vi "Create.vi"(7 "mode settings":variant, 8 "error in":errorcluster, 9 "number of default channels":i32, 10 "channel settings":variant, 11 "counter pwm input mode in":refnum<class "Counter PWM Input Mode.lvclass">) -> (0 "error out":errorcluster, 1 "channels":refnum<class "Channel.lvclass">[](array[class]), 3 "counter pwm input mode out":refnum<class "Counter PWM Input Mode.lvclass">)   [LabVIEW 2017, in "Counter PWM Input Mode.lvclass"]
uses:
  Counter PWM Input Mode.lvclass
  Channel Classes/Channel/Channel.lvclass
  Controls/counter pwm input channel settings.ctl
  Channel Classes/PWM Input Channel/Measurement Type.ctl
  f5685796-a93e-4056-970a-a8238cbbc772.vi
  Channel Classes/PWM Input Channel/PWM Input Channel.lvclass
  C:/dev/github.com/debryant/niveristand-scan-engine-ethercat-custom-device/Custom Device Source/Scripting/Modules/Channel Classes/Channel/Channel.lvclass
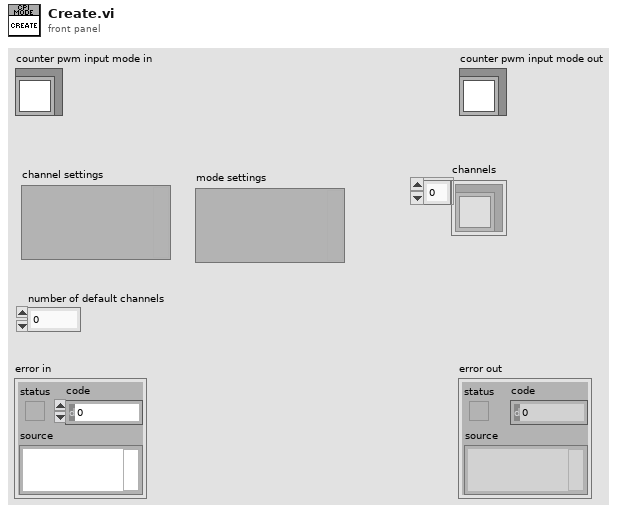
[diagram p1: front panel]
types:
  T1 = typedef "counter pwm input channel settings.ctl" = cluster{"name":string, "default value":dbl, "measurement type":T2}
  T2 = typedef "Scan Engine Scripting.lvlib/PWM Input Channel.lvclass/Measurement Type.ctl" = enum16{"High Pulse", "Low Pulse", "Most Recent"}
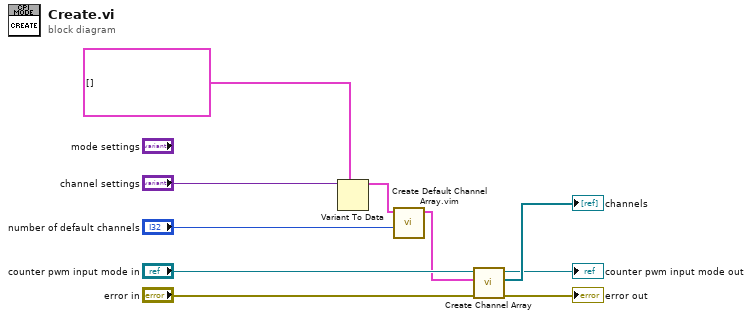
[diagram p0: block diagram]
diagram:
  n1 = Variant To Data(type=T1[] [], Variant="channel settings") -> (data=w8:T1[])  [unwired: 1 in, 1 out]
  n2 = call "Create Default Channel Array.vim"("number of default channels"="number of default channels", "channel settings in"=w8) -> ("channel settings out"=w1:T1[])  [unwired: 9 in]
  n3 = call "Create Channel Array.vi"("error in"="error in", "channel settings"=w1, "counter pwm input mode in"="counter pwm input mode in") -> ("error out"=→"error out":errorcluster, "channels"=→"channels":refnum<class "PWM Input Channel.lvclass">[], "counter pwm input mode out"=→"counter pwm input mode out":refnum<class "Counter PWM Input Mode.lvclass">)  [unwired: 6 in]
